vi "create.grid.vi"(8 "Origin":T1, 9 "Draw Area Size":T2, 10 "Plot End":timestamp, 11 "Plot Start":timestamp) -> (3 "picture":picture)   [LabVIEW 2024]
uses:
  <vilib>/Utility/miscctls.llb/LVBoundsTypeDef.ctl
  <vilib>/Utility/miscctls.llb/LVPointTypeDef.ctl
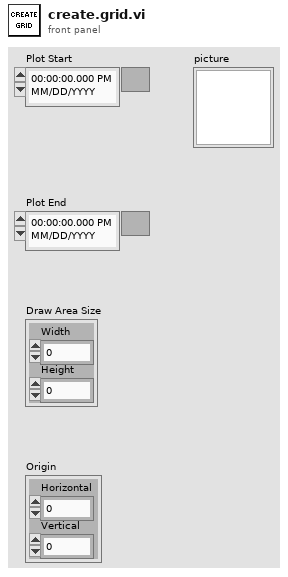
[diagram p1: front panel]
types:
  T1 = typedef "LVPointTypeDef.ctl" = cluster{"Horizontal":i16, "Vertical":i16}
  T2 = typedef "LVBoundsTypeDef.ctl" = cluster{"Width":u32, "Height":u32}
  T3 = cluster{"Width":u16, "Style":enum32{"Solid", "Dash", "Dot", "DashDot", "DashDotDot"}}
  T4 = enum16{"None", "Stacked", "Clockwise", "Counterclockwise"}
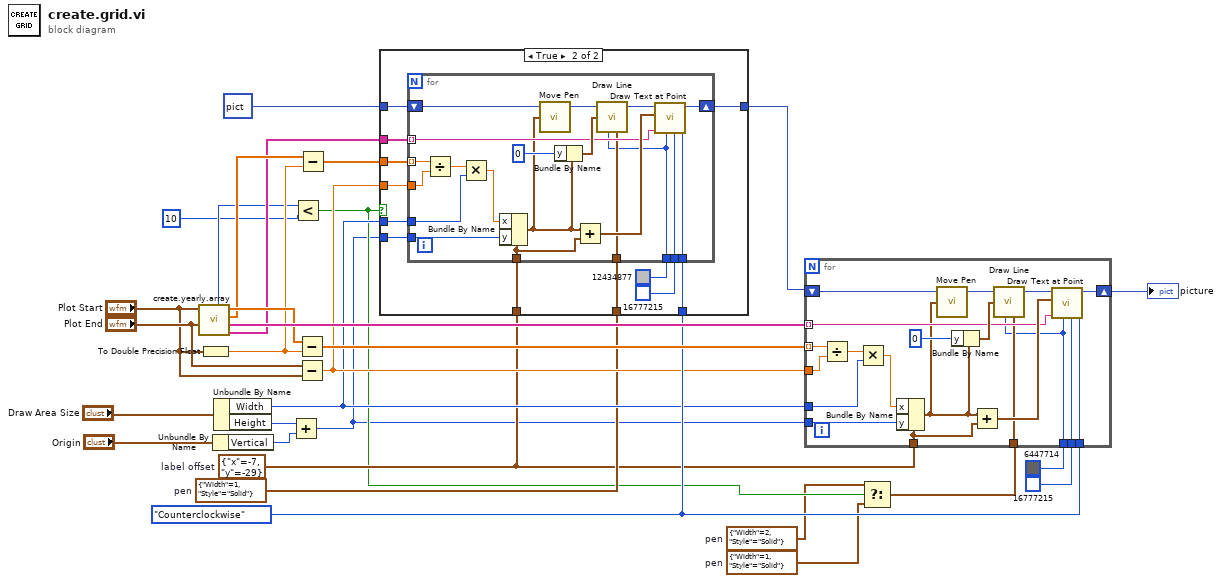
[diagram p0: block diagram]
diagram:
  w6 = T3 {"Width"=1, "Style"=enum."Solid"}  # pen
  w7 = T3 {"Width"=2, "Style"=enum."Solid"}  # pen
  w12 = T3 {"Width"=1, "Style"=enum."Solid"}  # pen
  w21 = T4."Counterclockwise" ("text orientation")
  w11 = cluster{"x":i16, "y":i16} {"x"=-7, "y"=-29}  # label offset
  n1 = call "create.yearly.array.vi"("end time"="Plot End", "start time"="Plot Start") -> ("month_names"=w15:string[], "year_names"=w25:string[], "month_timestamps"=w17:dbl[], "year_timestamps"=w22:dbl[], "years"=w10:i32)  [unwired: 5 in]
  n2 = To Double Precision Float(number="Plot Start") -> (double precision float=w16:dbl)
  n3 = Unbundle By Name("Origin") -> ("Vertical"=w2:i16)
  n4 = Unbundle By Name("Draw Area Size") -> ("Width"=w13:u32, "Height"=w3:u32)
  n5 = Add(x=w3, y=w2) -> (x+y=w1:u32)
  n6 = Less?(x=w10, y=10) -> (x < y?=w8:bool)
  n7 = Subtract(x=w22, y=w16) -> (x-y=w23:dbl[])
  n8 = Subtract(x="Plot End", y="Plot Start") -> (x-y=w14:dbl)
  n9 = Subtract(x=w17, y=w16) -> (x-y=w18:dbl[])
  n10 = case shown="True" w8 {
    tunnel: w21 -> [_ w43]
    tunnel: [w31 w42] -> w20
    tunnel: picture data[5B] ("picture") -> [w31 w41]
    tunnel: w18 -> [_ w40]
    tunnel: w15 -> [_ w39]
    tunnel: w14 -> [_ w38]
    tunnel: w13 -> [_ w37]
    tunnel: w1 -> [_ w36]
    tunnel: w12 -> [_ w33]
    tunnel: w11 -> [_ w32]
    frame False {
    }
    frame True {
      n11 = for {
        tunnel: w40 -> [w63] mode=indexing
        shift-right: [w56] -> w42
        shift-left: w41 -> [w55]
        tunnel: w38 -> [w62]
        tunnel: w37 -> [w60]
        tunnel: w36 -> [w59]
        tunnel: w39 -> [w51] mode=indexing
        tunnel: w43 -> [w50]
        tunnel: w33 -> [w49]
        tunnel: w32 -> [w46]
        tunnel: u32 16777215 ("BG color(transparent)") -> [w47]
        tunnel: u32 12434877 ("color(black)") -> [w45]
        n12 = Divide(x=w63, y=w62) -> (x/y=w61:dbl)
        n13 = Multiply(x=w61, y=w60) -> (x*y=w44:dbl)
        n14 = Bundle By Name(cluster=w46, "x"=w44, "y"=w59) -> (w48:cluster{"x":i16, "y":i16})
        n15 = call <vilib>:"Move Pen.vi"("new position"=w48, "picture"=w55) -> ("new picture"=w58:picture)  [unwired: 3 in]
        n16 = Bundle By Name(cluster=w48, "y"=i16 0) -> (w52:cluster{"x":i16, "y":i16})
        n17 = Add(x=w48, y=w46) -> (x+y=w54:cluster{"x":i16, "y":i16})
        n18 = call <vilib>:"Draw Line.vi"("picture"=w58, "end point"=w52, "color(black)"=w45, "pen"=w49) -> ("new picture"=w57:picture)  [unwired: 5 in]
        n19 = call <vilib>:"Draw Text at Point.vi"("text orientation"=w50, "BG color(transparent)"=w47, "text color(black)"=w45, "text"=w51, "origin"=w54, "picture"=w57) -> ("new picture"=w56:picture)  [unwired: 4 in, 1 out]
      }
    }
  }
  n20 = Select(t=w7, s=w8, f=w6) -> (s? t:f=w5:T3)
  n21 = for {
    tunnel: w23 -> [w83] mode=indexing
    shift-right: [w76] -> w26
    shift-left: w20 -> [w75]
    tunnel: w14 -> [w82]
    tunnel: w13 -> [w80]
    tunnel: w1 -> [w79]
    tunnel: w25 -> [w71] mode=indexing
    tunnel: w21 -> [w70]
    tunnel: w5 -> [w69]
    tunnel: w11 -> [w66]
    tunnel: u32 16777215 ("BG color(transparent)") -> [w67]
    tunnel: u32 6447714 ("color(black)") -> [w65]
    n22 = Divide(x=w83, y=w82) -> (x/y=w81:dbl)
    n23 = Multiply(x=w81, y=w80) -> (x*y=w64:dbl)
    n24 = Bundle By Name(cluster=w66, "x"=w64, "y"=w79) -> (w68:cluster{"x":i16, "y":i16})
    n25 = call <vilib>:"Move Pen.vi"("new position"=w68, "picture"=w75) -> ("new picture"=w78:picture)  [unwired: 3 in]
    n26 = Bundle By Name(cluster=w68, "y"=i16 0) -> (w72:cluster{"x":i16, "y":i16})
    n27 = Add(x=w68, y=w66) -> (x+y=w74:cluster{"x":i16, "y":i16})
    n28 = call <vilib>:"Draw Line.vi"("picture"=w78, "end point"=w72, "color(black)"=w65, "pen"=w69) -> ("new picture"=w77:picture)  [unwired: 5 in]
    n29 = call <vilib>:"Draw Text at Point.vi"("text orientation"=w70, "BG color(transparent)"=w67, "text color(black)"=w65, "text"=w71, "origin"=w74, "picture"=w77) -> ("new picture"=w76:picture)  [unwired: 4 in, 1 out]
  }
  "picture" <- w26
